vi "LVCAM Create Nest.vi"(9 "Alias":string, 10 "Nest Actor":refnum<class "LVCAM.lvclass">, 11 "LVCAM Create Nest in":refnum<class "LVCAM Create Nest.lvclass">) -> (0 "error out":errorcluster, 3 "LVCAM Create Nest out":refnum<class "LVCAM Create Nest.lvclass">)   [LabVIEW 2021, in "LVCAM Create Nest.lvlib" / "LVCAM Create Nest.lvclass"]
uses:
  LVCAM Create Nest.lvclass
  LVCAM/LVCAM/LVCAM.lvclass
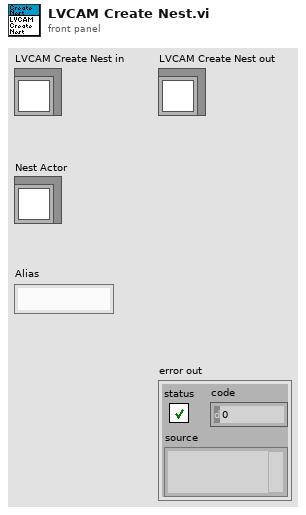
[diagram p1: front panel]
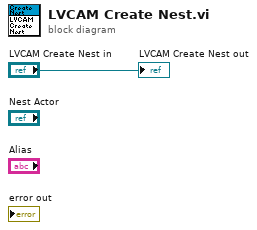
[diagram p0: block diagram]
diagram:
  "LVCAM Create Nest out" <- "LVCAM Create Nest in"
